vi "BiStateVariableToggle Example.vi"() -> ()   [LabVIEW 2017]
uses:
  Global State Variables.vi
panel:
  in  "stop":bool
  in  "State Selector Methods":T1(tab)=enum."test single button vi"
  in  "single buton selector":bool
  in  "right button\nselector":bool
  in  "left button \nselector":bool
  in  "Test Single Button vi":bool
  in  "Test Single Button vi 2":bool
  in  "Test Single Button vi 5":bool
  in  "Test Single Button vi 6":bool
  in  "Button 2":bool
  in  "Button 1":bool
  in  "Button 3":bool
  in  "Button 4":bool
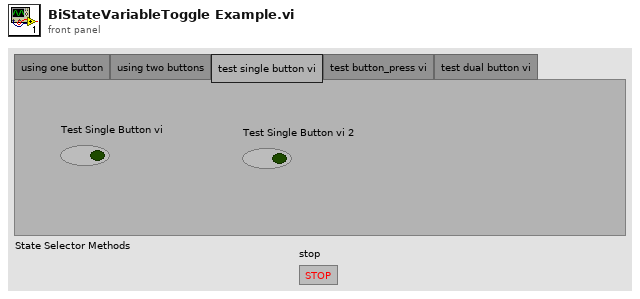
[diagram p1: front panel]
types:
  T1 = enum32{"using one button", "using two buttons", "test single button vi", "test button_press vi", "test dual button vi"}
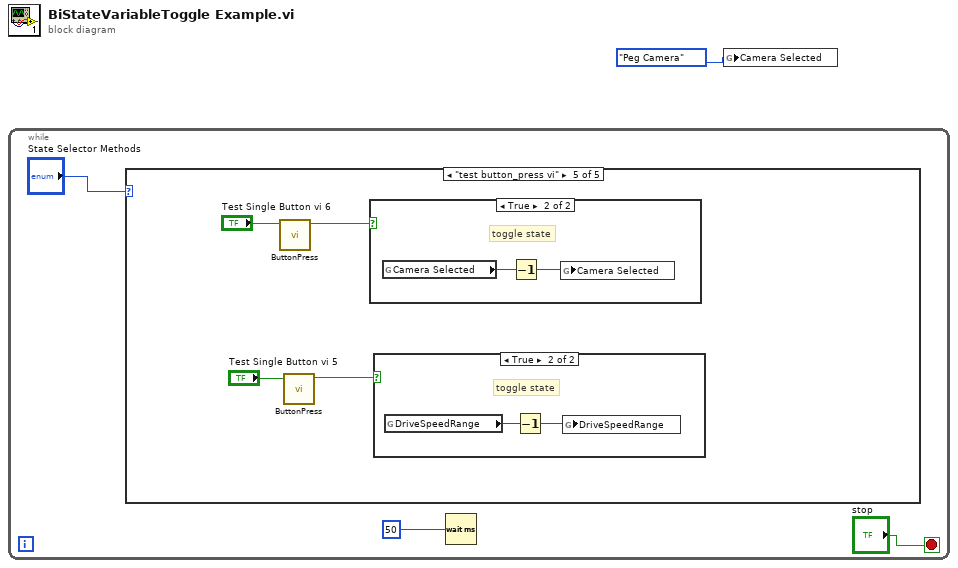
[diagram p0: block diagram]
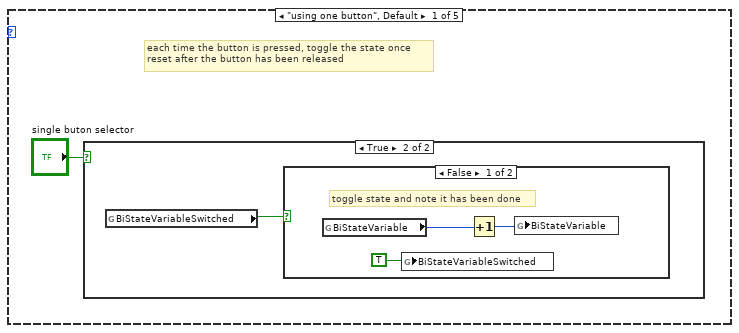
[diagram p2: hidden frame]
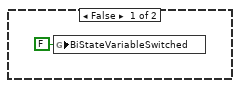
[diagram p3: hidden frame]
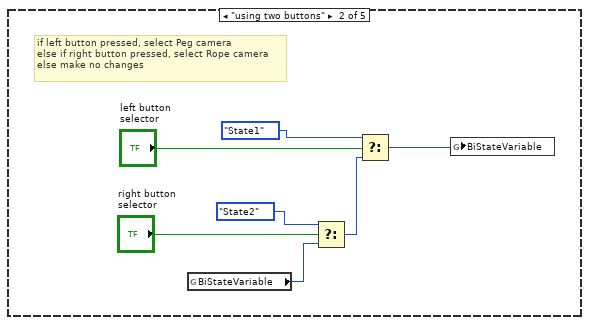
[diagram p5: hidden frame]
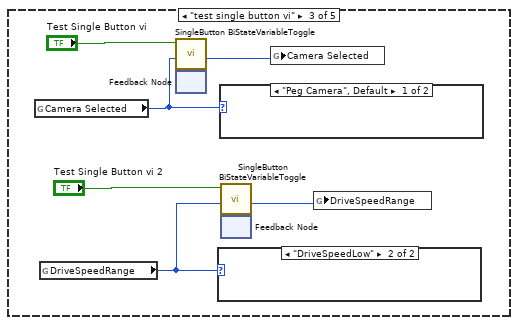
[diagram p6: hidden frame]
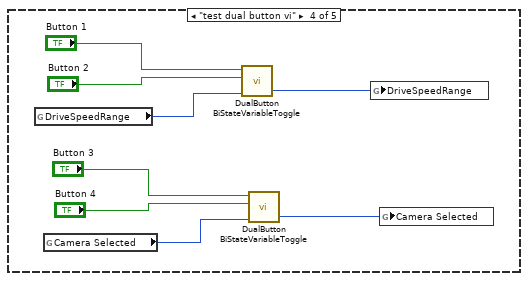
[diagram p9: hidden frame]
diagram:
  n1 = while {
    stop <- "stop" stop-if-true
    n2 = case shown="\"test button_press vi\"" "State Selector Methods" {
      frame "using one button", Default {
        # "each time the button is pressed, toggle the state once \nreset after the button has been released"
        n3 = case shown="True" "single buton selector" {
          frame False {
            n4 = global write "Global State Variables.vi" "BiStateVariableSwitched"(FALSE ("BiStateVariableToggle")) -> ()
          }
          frame True {
            n5 = global read "Global State Variables.vi" "BiStateVariableSwitched"() -> (w7:bool)
            n6 = case shown="False" w7 {
              frame False {
                # "toggle state and note it has been done"
                n7 = global read "Global State Variables.vi" "BiStateVariable"() -> (w10:enum16{"State1", "State2"})
                n8 = global write "Global State Variables.vi" "BiStateVariableSwitched"(TRUE ("BiStateVariableToggle")) -> ()
                n9 = Increment(x=w10) -> (x+1=w9:enum16{"State1", "State2"})
                n10 = global write "Global State Variables.vi" "BiStateVariable"(w9) -> ()
              }
              frame True {
                # "state already been switched"
              }
            }
          }
        }
      }
      frame "using two buttons" {
        # "if left button pressed, select Peg camera\nelse if right button pressed, select Rope camera\nelse make no changes"
        n11 = global read "Global State Variables.vi" "BiStateVariable"() -> (w13:enum16{"State1", "State2"})
        n12 = Select(t=enum16{"State1", "State2"}."State2", s="right button\nselector", f=w13) -> (s? t:f=w15:enum16{"State1", "State2"})
        n13 = Select(t=enum16{"State1", "State2"}."State1", s="left button \nselector", f=w15) -> (s? t:f=w16:enum16{"State1", "State2"})
        n14 = global write "Global State Variables.vi" "BiStateVariable"(w16) -> ()
      }
      frame "test single button vi" {
        n15 = global read "Global State Variables.vi" "Camera Selected"() -> (w20:enum16{"Peg Camera", "Rope Camera"})
        n16 = global read "Global State Variables.vi" "DriveSpeedRange"() -> (w25:enum16{"DriveSpeedHigh", "DriveSpeedLow"})
        n17 = feedback #1() -> (w18:bool)  [unwired: 1 in]
        n18 = call "SingleButton BiStateVariableToggle.vi"("AlreadySwitched?"=w18, "PreviousState"=w20, "Button"="Test Single Button vi") -> ("NewState"=w21:u16, "StillSwitched?"=w19:bool)  [unwired: 7 in]
        n19 = feedback-in #1(w19) -> ()
        n20 = case shown="\"DriveSpeedLow\"" w25 {
          frame "DriveSpeedHigh", Default {
          }
          frame "DriveSpeedLow" {
          }
        }
        n21 = case shown="\"Peg Camera\", Default" w20 {
          frame "Peg Camera", Default {
          }
          frame "Rope Camera" {
          }
        }
        n22 = feedback #2() -> (w23:bool)  [unwired: 1 in]
        n23 = call "SingleButton BiStateVariableToggle.vi"("AlreadySwitched?"=w23, "PreviousState"=w25, "Button"="Test Single Button vi 2") -> ("NewState"=w26:u16, "StillSwitched?"=w24:bool)  [unwired: 7 in]
        n24 = feedback-in #2(w24) -> ()
        n25 = global write "Global State Variables.vi" "Camera Selected"(w21) -> ()
        n26 = global write "Global State Variables.vi" "DriveSpeedRange"(w26) -> ()
      }
      frame "test dual button vi" {
        n27 = global read "Global State Variables.vi" "DriveSpeedRange"() -> (w32:enum16{"DriveSpeedHigh", "DriveSpeedLow"})
        n28 = global read "Global State Variables.vi" "Camera Selected"() -> (w28:enum16{"Peg Camera", "Rope Camera"})
        n29 = call "DualButton BiStateVariableToggle.vi"("PreviousState"=w32, "ButtonToSelect\nSecondState"="Button 2", "ButtonToSelect\nFirstState"="Button 1") -> ("NewState"=w33:u16)  [unwired: 8 in]
        n30 = call "DualButton BiStateVariableToggle.vi"("PreviousState"=w28, "ButtonToSelect\nSecondState"="Button 4", "ButtonToSelect\nFirstState"="Button 3") -> ("NewState"=w29:u16)  [unwired: 8 in]
        n31 = global write "Global State Variables.vi" "DriveSpeedRange"(w33) -> ()
        n32 = global write "Global State Variables.vi" "Camera Selected"(w29) -> ()
      }
      frame "test button_press vi" {
        n33 = call "ButtonPress.vi"("Button In"="Test Single Button vi 6") -> ("Button Pressed?"=w38:bool)  [unwired: 10 in]
        n34 = call "ButtonPress.vi"("Button In"="Test Single Button vi 5") -> ("Button Pressed?"=w37:bool)  [unwired: 10 in]
        n35 = case shown="True" w38 {
          frame False {
          }
          frame True {
            # "toggle state"
            n36 = global read "Global State Variables.vi" "Camera Selected"() -> (w43:enum16{"Peg Camera", "Rope Camera"})
            n37 = Decrement(x=w43) -> (x-1=w42:enum16{"Peg Camera", "Rope Camera"})
            n38 = global write "Global State Variables.vi" "Camera Selected"(w42) -> ()
          }
        }
        n39 = case shown="True" w37 {
          frame False {
          }
          frame True {
            # "toggle state"
            n40 = global read "Global State Variables.vi" "DriveSpeedRange"() -> (w41:enum16{"DriveSpeedHigh", "DriveSpeedLow"})
            n41 = Decrement(x=w41) -> (x-1=w40:enum16{"DriveSpeedHigh", "DriveSpeedLow"})
            n42 = global write "Global State Variables.vi" "DriveSpeedRange"(w40) -> ()
          }
        }
      }
    }
    n43 = Wait (ms)(milliseconds to wait=u32 50) -> ()  [unwired: 1 out]
  }
  n44 = global write "Global State Variables.vi" "Camera Selected"(enum16{"Peg Camera", "Rope Camera"}."Peg Camera" ("Camera Selected")) -> ()
